vi "myRIO_BRig_RT_dataLC_Selection_Probability_Switch_l1.vi"() -> (2 "output_Selection_Probability_Switch_l1":i32)   [LabVIEW 2014]
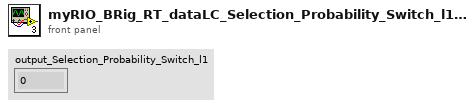
[diagram p1: front panel]
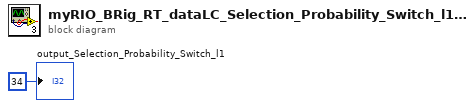
[diagram p0: block diagram]
diagram:
  "output_Selection_Probability_Switch_l1" <- 34 ("output_iBlock")
